vi "GetAllStringsInVIs.vi"() -> ()   [LabVIEW 2014]
panel:
  in  "Path":path=path "F:/TSBuild51/App/TestStandPublic/AdapterSupport/LabVIEW"
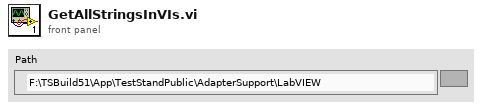
[diagram p1: front panel]
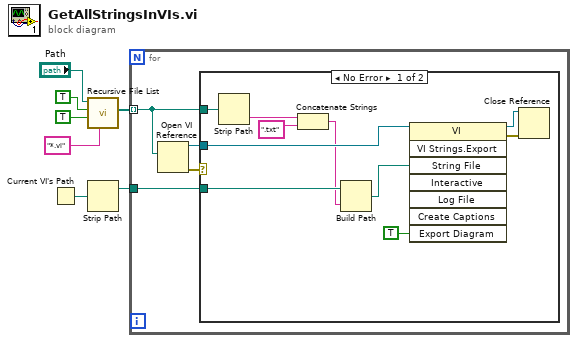
[diagram p0: block diagram]
diagram:
  n1 = Current VI's Path() -> (path=w1:path)
  n2 = call <vilib>:"Recursive File List.vi"("pattern"="*.vi", "Continue Recursing on Error? (F)"=TRUE, "Treat LLBs as Folders?"=TRUE, "Folder Path"="Path") -> ("All Files in Dir"=w4:path[])  [unwired: 1 in, 6 out]
  n3 = Strip Path(path=w1) -> (stripped path=w2:path)  [unwired: 1 out]
  n4 = for {
    tunnel: w4 -> [w8] mode=indexing
    tunnel: w2 -> [w9]
    n5 = Open VI Reference(vi path=w8) -> (vi reference=w10:refnum<vi>, error out=w11:errorcluster)  [unwired: 5 in]
    n6 = case shown="No Error" w11 {
      tunnel: w10 -> [w21 _]
      tunnel: w9 -> [w18 _]
      tunnel: w8 -> [w19 _]
      frame No Error {
        n7 = Strip Path(path=w19) -> (name=w17:string)  [unwired: 1 out]
        n8 = Concatenate Strings(w17, ".txt" ("string")) -> (w15:string)
        n9 = Build Path(base path=w18, name or relative path=w15) -> (appended path=w14:path)
        n10 = invoke class="VI" method="VI Strings.Export"(reference=w21, "String File"=w14, "Export Diagram"=TRUE) -> (reference out=w12:refnum<vi>, error out=w13:errorcluster)  [unwired: 5 in, 6 out]
        n11 = Close Reference(reference=w12, error in (no error)=w13) -> ()  [unwired: 1 out]
      }
      frame Error {
      }
    }
  }
